vi "FPGA Main.vi"() -> ()   [LabVIEW 2015]
uses:
  Type/_RW Status.ctl
  Type/_LED States.ctl
  Type/_FPGA States.ctl
  <vilib>/Platform/TimedLoop/XDataNode/timing_clust.ctl
  <vilib>/Platform/TimedLoop/XDataNode/nitl_modes.ctl
  <vilib>/Platform/TimedLoop/XDataNode/wakeup.ctl
  Type/_FPGA DC Lines.ctl
  <vilib>/rvi/Emulation/niFpgaGetClockAttributes.vi
  <vilib>/rvi/Emulation/niFpgaSctlEmulationGetInTimedLoop.vi
  <vilib>/rvi/Emulation/niFpgaEmulationReportErrorSimple.vi
  <vilib>/rvi/eio/common/nirviEmuTemplateMethod_errors.vi
  <vilib>/rvi/Emulation/niFpgaCriticalErrorInLSC.vi
  <vilib>/rvi/Emulation/niFpgaEmulationIsFPGAContextNoSignature.vi
  <vilib>/rvi/DataTransferAndStorage/Container/Common/niFpgaContainerGetUniqueNameForEmu.vi
  <vilib>/rvi/Memory/Memory_Emulation/niFpgaMemoryEmulationCacheClearOnFirstRun.vi
  <vilib>/rvi/Memory/Memory_Emulation/nirvimemoryEmulationManagerCache_MakeExclusive.vi
  <vilib>/rvi/Memory/Memory_Emulation/niFpgaMemoryEmulationValidateCache.vi
  <vilib>/rvi/Memory/Memory_Emulation/nirvimemoryEmulationManagerCache_InsertValue.vi
  <vilib>/Utility/error.llb/Clear Errors.vi
  <vilib>/rvi/Memory/Memory_Emulation/nirvimemoryEmulationManagerCache_ReleaseExclusive.vi
  <vilib>/rvi/Memory/Memory_Emulation/nirvimemoryEmulationManagerCache_GetValue.vi
  <vilib>/rvi/Memory/Memory_Emulation/nirvimemoryEmulationManagerCache_SetValue.vi
  <vilib>/rvi/Emulation/niFpgaProcessEmulError.vi
  <vilib>/rvi/Memory/Memory_Emulation/nirvimemoryEmulation.vi
  <vilib>/rvi/Memory/Memory_Emulation/nirvimemoryFastEmulation.vi
  <vilib>/rvi/Emulation/niFpgaSctlEmulationResourceMgr.vi
  <vilib>/rvi/errors/nirviReportUnexpectedCaseInternalError (U32).vi
  Instance           1 17Saved   FPGA Main .vi
  Instance           2 17Saved   FPGA Main .vi
  <vilib>/rvi/interface/RandomDataEmulation/niFpgaRandomDataHandleErrors.vi
  <vilib>/eio/EIONode/EIONode.xnode
  <vilib>/Platform/TimedLoop/XDataNode/XDataNode.xnode
  <vilib>/rvi/DataTransferAndStorage/Container/XNode/niFpgaContainer.xnode
  <vilib>/rvi/DataTransferAndStorage/Register/Emulation/niFpgaRegisterEmulation.vi
  <vilib>/rvi/interface/RandomDataEmulation/nirviRandomDataFpgaReadWriteTemplate.vi
  <vilib>/Platform/TimedLoop/XDataNode/XDNodeRunTimeDep.lvlib
panel:
  out "i":i32
  out "Run Mode":u8
  out "FPGA States":T1
  out "Acquiring Data":bool
  out "Ready to Acquire Data":bool
  out "LC Input Detected":bool
  out "Run In Progress":bool
  in  "ForceStart":bool
  in  "FilaB":bool
  in  "FilaC":bool
  in  "Send Serial":bool
  in  "Repeat":bool
  in  "LED States":T2
  in  "Update":bool
  out "Version":u32
  in  "R/W Status":T3
  in  "Start":bool
  out "Running":bool
  in  "Address":u16
  in  "Data":u32
  in  "Read/Write":bool
  # "Memory Map Access"
  # "Run Cycle Control"
  # "VG Filament Control"
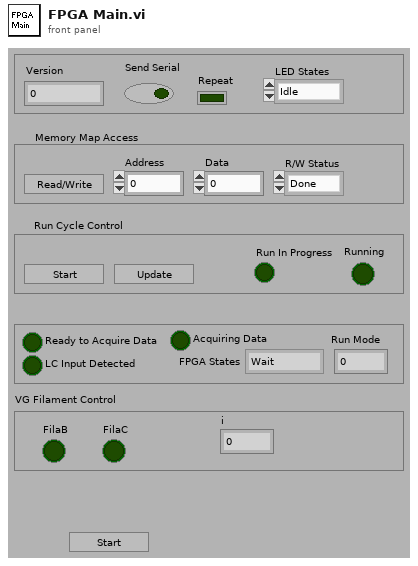
[diagram p1: front panel]
types:
  T1 = typedef "_FPGA States.ctl" = enum8{"Wait", "Single", "Dual", "DoCycles", "RampParam", "ReadADC", "SetOscil", "SetPIC", "EleOn", "Stop"}
  T2 = typedef "_LED States.ctl" = enum8{"Idle", "Solid B", "Solid R", "Solid P", "Off B", "Off R", "Off P", "Off BRP", "Off RP", "Flash R&P", "Flash P"}
  T3 = typedef "_RW Status.ctl" = enum8{"Done", "Do Read", "Do Write", "Set Latch1", "Set Latch2", "Set Latch3", "Set Latch4", "RP ON", "EL ON", "Serial Send", "Set LC Out", "Get LC In", "Read VAC", "Table Test", "Get Interlock", "Do Read2", "Do Write2"}
  T4 = typedef "_FPGA DC Lines.ctl" = enum16{"Q1 POL", "Q3 POL", "Q1 DC EN", "Q3 DC EN", "COR POL", "CUR POL", "S1 POL", "S2 POL", "CEM POL"}
  T5 = typedef "XDNodeRunTimeDep.lvlib/timing_clust.ctl" = cluster{"Expected End [f-1]":u64, "Actual End [f-1]":u64, "Finished Late? [f-1]":bool, "Expected End [i-1]":u64, "Actual End [i-1]":u64, "Finished Late? [i-1]":bool, "Expected Start [i]":u64, "Actual Start [i]":u64, "Expected Start [f]":u64, "Actual Start [f]":u64, "Source Name":string, "Structure Name":string, "Period":i64, "Deadline":i64, "Offset":i64, "Start":i64, "Priority":i32, "Timeout":i32, "Mode":T6, "Wakeup Reason":T7, "Error":errorcluster, "Source Type":string, "Secondary Source Type":string, "Global End Time":u64, "Global Start Time":u64, "Frame Duration":u64, "Iteration Duration":u64, "Assigned CPU":i32, "I/O Scan Engine Mode":u32}
  T6 = typedef "XDNodeRunTimeDep.lvlib/nitl_modes.ctl" = enum32{"No Change", "Process missed periods, maintain original phase", "Discard missed periods, maintain original phase", "Process missed periods, ignore original phase", "Discard missed periods, ignore original phase"}
  T7 = typedef "XDNodeRunTimeDep.lvlib/wakeup.ctl" = enum32{"Normal", "Aborted", "Asynchronous wakeup", "Timing source error", "Timed loop error", "Timeout"}
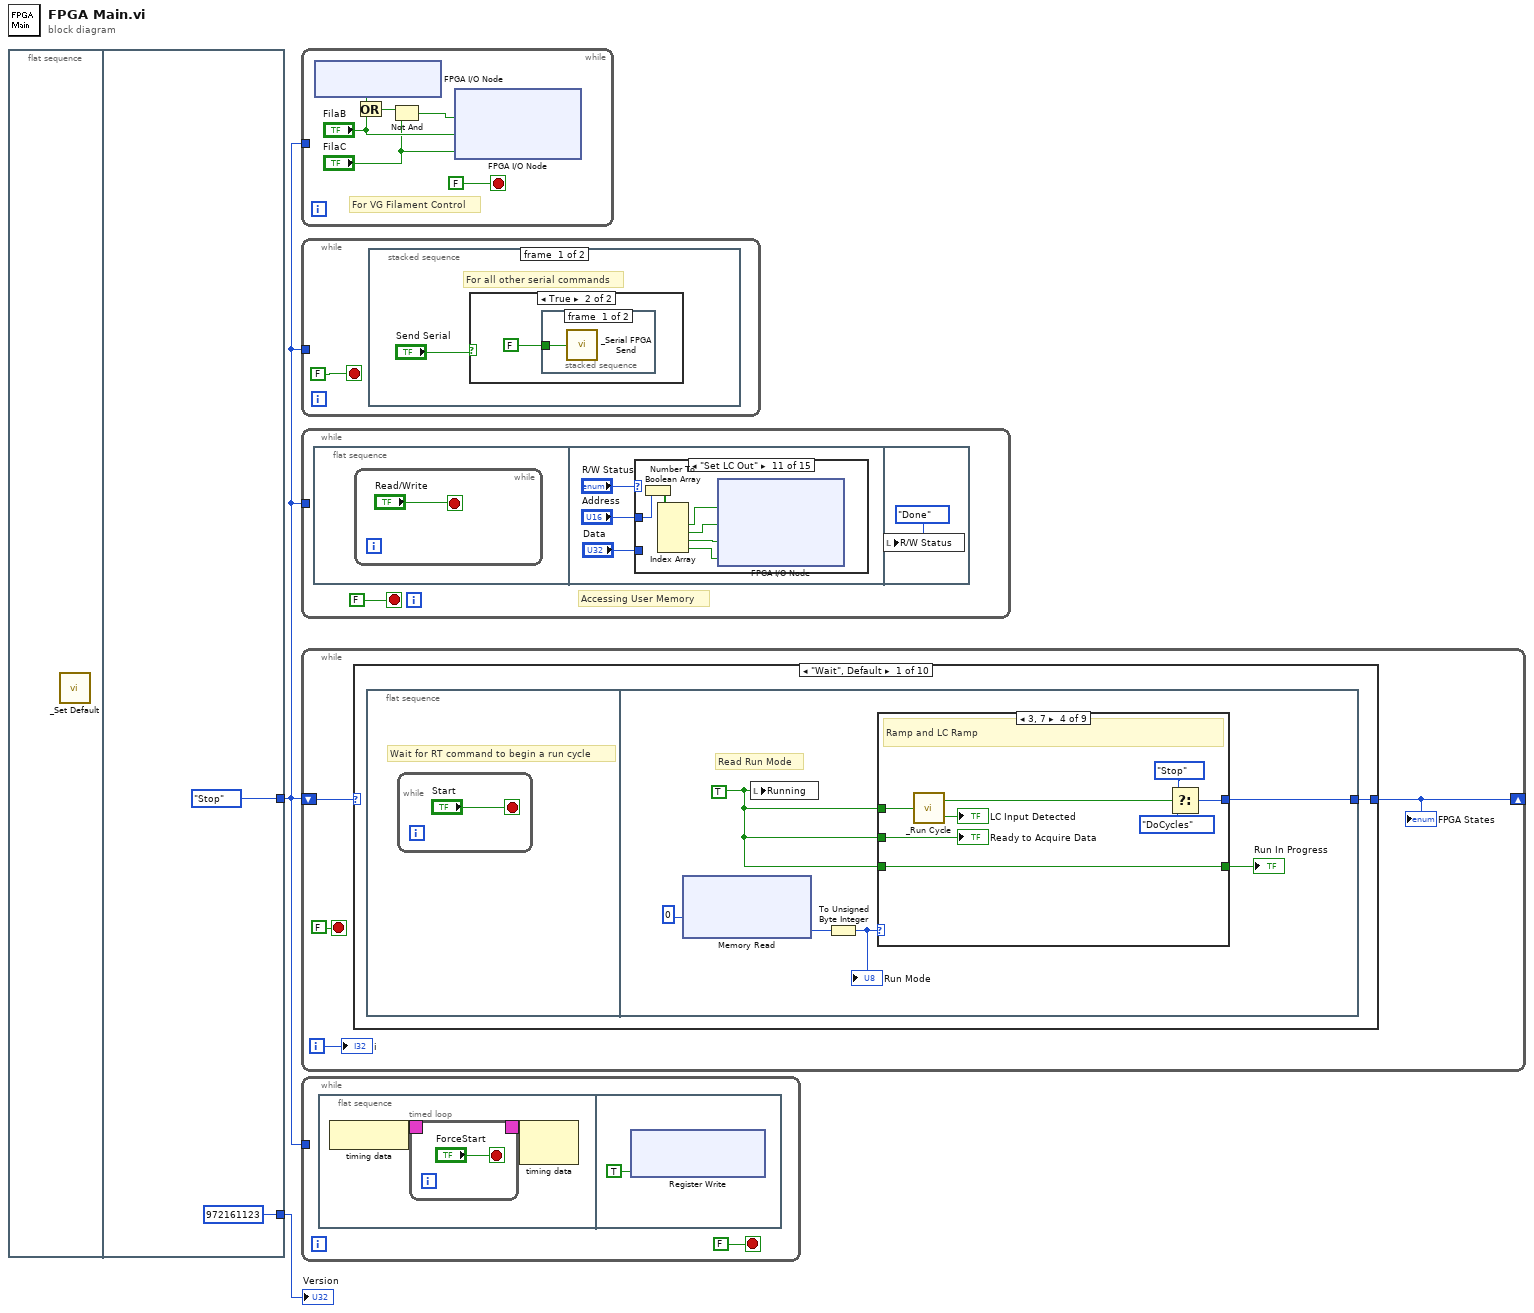
[diagram p0: block diagram]
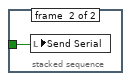
[diagram p3: hidden frame]
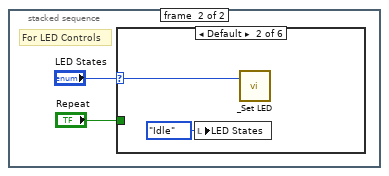
[diagram p4: hidden frame]
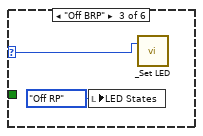
[diagram p6: hidden frame]
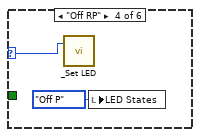
[diagram p7: hidden frame]
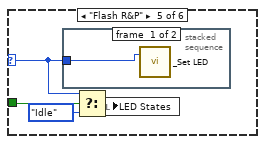
[diagram p8: hidden frame]
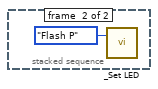
[diagram p9: hidden frame]
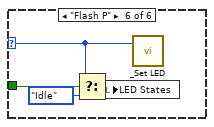
[diagram p10: hidden frame]
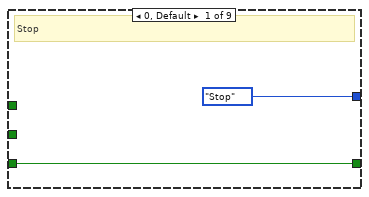
[diagram p11: hidden frame]
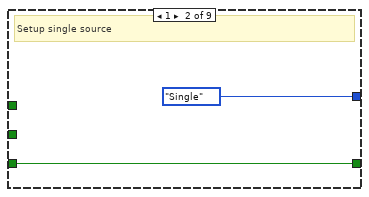
[diagram p12: hidden frame]
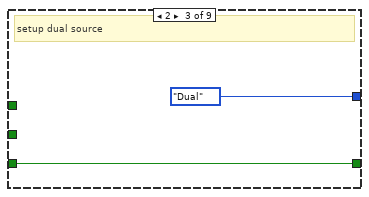
[diagram p13: hidden frame]
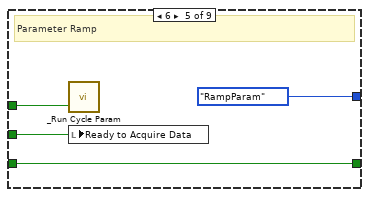
[diagram p14: hidden frame]
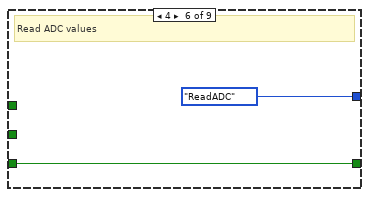
[diagram p15: hidden frame]
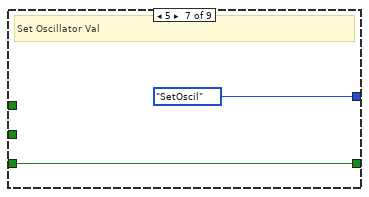
[diagram p16: hidden frame]
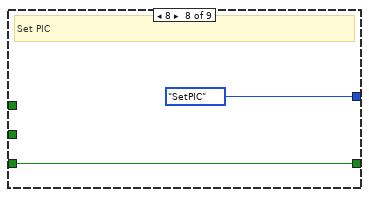
[diagram p17: hidden frame]
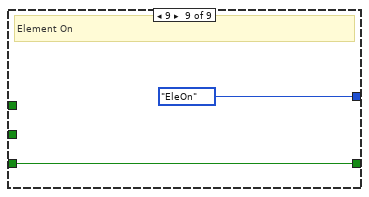
[diagram p18: hidden frame]
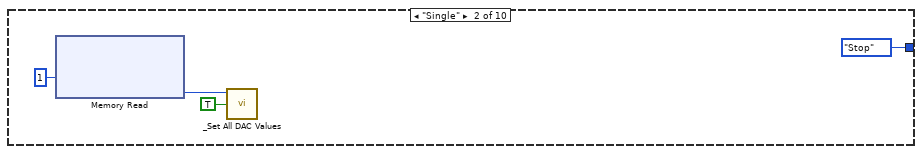
[diagram p19: hidden frame]
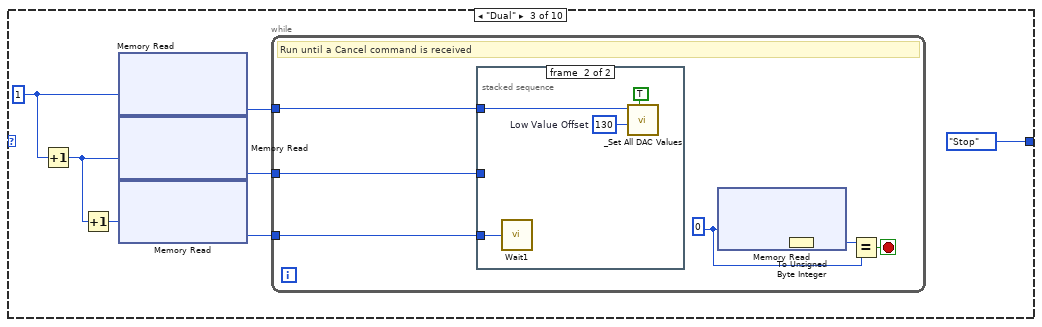
[diagram p20: hidden frame]
diagram:
  n1 = flat-sequence {
    tunnel: [_FPGA_States."Stop" ("FPGA States")] -> w2
    tunnel: [u32 972161123 ("Version")] -> w1
    frame #0 {
      n2 = call "_Set Default.vi"() -> ()  [unwired: 6 out]
    }
    frame #1 {
    }
  }
  n3 = while {
    tunnel: w2 -> [_]
    stop <- FALSE stop-if-true
    # "For VG Filament Control"
    n4 = xnode "FPGA I/O Node"() -> ("Digtal IO/DIO65"=w9:bool)  [unwired: 1 in, 1 out]
    n5 = Or(x=w9, y="FilaB") -> (x .or. y?=w8:bool)
    n6 = Not And(1:"FilaC", 2:w8) -> (0:w7:bool)
    n7 = xnode "FPGA I/O Node"("Digtal IO/DIO68"=w7, "Digtal IO/DIO66"="FilaB", "Digtal IO/DIO67"="FilaC") -> ()  [unwired: 3 in, 3 out]
  }
  n8 = while {
    tunnel: w2 -> [_]
    stop <- FALSE stop-if-true
    n9 = stacked-sequence {
      frame #0 {
        # "For all other serial commands"
        n10 = case shown="True" "Send Serial" {
          frame False {
          }
          frame True {
            n11 = stacked-sequence {
              tunnel: FALSE ("LED Control (T)") -> [w14 w15]
              frame #0 {
                n12 = call "_Serial FPGA Send.vi"("LED Control (T)"=w14) -> ()
              }
              frame #1 {
                n13 = local write "Send Serial"(w15) -> ()
              }
            }
          }
        }
      }
      frame #1 {
        # "For LED Controls"
        n14 = case shown="Default" "LED States" {
          selector: "LED States" -> [_ w18 w20 w22 w24 w30]
          tunnel: "Repeat" -> [_ _ _ _ w27 w33]
          frame "Idle" {
          }
          frame Default {
            n15 = local write "LED States"(_LED_States."Idle" ("LED States")) -> ()
            n16 = call "_Set LED.vi"("LED States"=w18) -> ()  [unwired: 3 out]
          }
          frame "Off BRP" {
            n17 = local write "LED States"(_LED_States."Off RP" ("LED States")) -> ()
            n18 = call "_Set LED.vi"("LED States"=w20) -> ()  [unwired: 3 out]
          }
          frame "Off RP" {
            n19 = call "_Set LED.vi"("LED States"=w22) -> ()  [unwired: 3 out]
            n20 = local write "LED States"(_LED_States."Off P" ("LED States")) -> ()
          }
          frame "Flash R&P" {
            n21 = stacked-sequence {
              tunnel: w24 -> [w28 _]
              frame #0 {
                n22 = call "_Set LED.vi"("LED States"=w28) -> ()  [unwired: 3 out]
              }
              frame #1 {
                n23 = call "_Set LED.vi"("LED States"=_LED_States."Flash P") -> ()  [unwired: 3 out]
              }
            }
            n24 = Select(t=w24, s=w27, f=_LED_States."Idle") -> (s? t:f=w26:T2)
            n25 = local write "LED States"(w26) -> ()
          }
          frame "Flash P" {
            n26 = Select(t=w30, s=w33, f=_LED_States."Idle") -> (s? t:f=w32:T2)
            n27 = local write "LED States"(w32) -> ()
            n28 = call "_Set LED.vi"("LED States"=w30) -> ()  [unwired: 3 out]
          }
        }
      }
    }
  }
  n29 = while {
    tunnel: w2 -> [_]
    stop <- FALSE stop-if-true
    # "Accessing User Memory"
    n30 = flat-sequence {
      frame #0 {
        n31 = while {
          stop <- "Read/Write" stop-if-true
        }
      }
      frame #1 {
        n32 = case shown="\"Set LC Out\"" "R/W Status" {
          tunnel: "Address" -> [_ w39 w42 w44 w46 w47 w49 w51 w53 w55 w61 _ _ _ _]
          tunnel: "Data" -> [_ _ _ w43 w45 _ _ _ _ _ _ _ _ _ _]
          frame "Done", Default {
          }
          frame "Do Read" {
            n33 = xnode ("Memory Read")("Address"=w39) -> ("Data"=w40:u32)  [unwired: 1 in, 1 out]
            n34 = local write "Data"(w40) -> ()
          }
          frame "Do Read2" {
            n35 = xnode ("Memory Read")("Address"=w42) -> ("Data"=w41:u32)  [unwired: 1 in, 1 out]
            n36 = local write "Data"(w41) -> ()
          }
          frame "Do Write" {
            n37 = xnode ("Memory Write")("Address"=w44, "Data"=w43) -> ()  [unwired: 1 in, 1 out]
          }
          frame "Do Write2" {
            n38 = xnode ("Memory Write")("Address"=w46, "Data"=w45) -> ()  [unwired: 1 in, 1 out]
          }
          frame "Set Latch1" {
            n39 = call "_Set DC Line.vi"("States"=w47, "DC Line"=_FPGA_DC_Lines."Q1 POL") -> ()  [unwired: 2 out]
          }
          frame "Set Latch2" {
            n40 = call "_Set DC Line.vi"("States"=w49, "DC Line"=_FPGA_DC_Lines."COR POL") -> ()  [unwired: 2 out]
          }
          frame "Set Latch3" {
            n41 = call "_Set DC Line.vi"("States"=w51, "DC Line"=_FPGA_DC_Lines."S1 POL") -> ()  [unwired: 2 out]
          }
          frame "Set Latch4" {
            n42 = call "_Set DC Line.vi"("States"=w53, "DC Line"=_FPGA_DC_Lines."CEM POL") -> ()  [unwired: 2 out]
          }
          frame "RP ON" {
            n43 = Greater Than 0?(x=w55) -> (x > 0?=w56:bool)
            n44 = xnode "FPGA I/O Node"("Digtal IO/DIO18"=w56) -> ()  [unwired: 1 in, 1 out]
          }
          frame "Set LC Out" {
            n45 = Number To Boolean Array(number=w61) -> (Boolean array=w62:bool[])
            n46 = Index Array(array=w62) -> (element #1=w60:bool, element #2=w59:bool, element #3=w58:bool, element #4=w57:bool)  [unwired: 4 in]
            n47 = xnode "FPGA I/O Node"("Digtal IO/DIO49"=w60, "Digtal IO/DIO50"=w59, "Digtal IO/DIO52"=w58, "Digtal IO/DIO56"=w57) -> ()  [unwired: 4 in, 4 out]
          }
          frame "Get LC In" {
            # "LC2-I1"
            # "LC1-I1"
            n48 = xnode "FPGA I/O Node"() -> ("Digtal IO/DIO51"=w67:bool, "Digtal IO/DIO53"=w66:bool)  [unwired: 2 in, 2 out]
            n49 = Boolean To (0,1)(Boolean=w66) -> (0, 1=w64:i16)
            n50 = Boolean To (0,1)(Boolean=w67) -> (0, 1=w65:i16)
            n51 = Join Numbers(hi=w65, lo=w64) -> ((hi.lo)=w63:u32)
            n52 = local write "Data"(w63) -> ()
          }
          frame "Get Interlock" {
            # "Card cage door"
            n53 = xnode "FPGA I/O Node"() -> ("Digtal IO/DIO60"=w69:bool)  [unwired: 1 in, 1 out]
            n54 = Boolean To (0,1)(Boolean=w69) -> (0, 1=w68:i16)
            n55 = local write "Data"(w68) -> ()
          }
          frame "Read VAC" {
            n56 = call "_Read VAC Gauge.vi"() -> ("DAC"=w70:u8)
            n57 = local write "Data"(w70) -> ()
          }
          frame "Table Test" {
            n58 = call "_Table Test.vi"() -> ()  [unwired: 1 out]
          }
        }
      }
      frame #2 {
        n59 = local write "R/W Status"(_RW_Status."Done" ("RW Status")) -> ()
      }
    }
  }
  n60 = while {
    shift-right: [w74] -> _
    shift-left: w2 -> [w75]
    i -> [w72]
    stop <- FALSE stop-if-true
    n61 = case shown="\"Wait\", Default" w75 {
      tunnel: [w76 _FPGA_States."Stop" ("FPGA States") _FPGA_States."Stop" ("FPGA States") _FPGA_States."Stop" ("FPGA States") _FPGA_States."Stop" ("FPGA States") _FPGA_States."Stop" ("FPGA States") _FPGA_States."Stop" ("FPGA States") _FPGA_States."Stop" ("FPGA States") _FPGA_States."Stop" ("FPGA States") _FPGA_States."Wait" ("FPGA States")] -> w74
      frame "Wait", Default {
        n62 = flat-sequence {
          tunnel: [w83] -> w76
          frame #0 {
            # "Wait for RT command to begin a run cycle"
            n63 = while {
              stop <- "Start" stop-if-true
            }
          }
          frame #1 {
            w78 = TRUE ("Running")
            # "Read Run Mode"
            n64 = xnode ("Memory Read")("Address"=u8 0) -> ("Data"=w82:u32)  [unwired: 1 in, 1 out]
            n65 = local write "Running"(w78) -> ()
            n66 = To Unsigned Byte Integer(number=w82) -> (unsigned 8bit integer=w80:u8)
            "Run Mode" <- w80
            n67 = case shown="3, 7" w80 {
              tunnel: [_FPGA_States."Stop" ("FPGA States") _FPGA_States."Single" ("FPGA States") _FPGA_States."Dual" ("FPGA States") w94 _FPGA_States."RampParam" ("FPGA States") _FPGA_States."ReadADC" ("FPGA States") _FPGA_States."SetOscil" ("FPGA States") _FPGA_States."SetPIC" ("FPGA States") _FPGA_States."EleOn" ("FPGA States")] -> w83
              tunnel: w78 -> [_ _ _ w93 w100 _ _ _ _]
              tunnel: [w84 w86 w88 w92 w99 w102 w104 w106 w108] -> w79
              tunnel: w78 -> [w84 w86 w88 w92 w99 w102 w104 w106 w108]
              tunnel: w78 -> [_ _ _ w90 w98 _ _ _ _]
              frame 0, Default {
                # "Stop"
              }
              frame 1 {
                # "Setup single source"
              }
              frame 2 {
                # "setup dual source"
              }
              frame 3, 7 {
                # "Ramp and LC Ramp"
                n68 = call "_Run Cycle.vi"("Init (F)"=w93) -> ("LC Input Detected"=→"LC Input Detected":bool, "Finish Run?"=w97:bool)  [unwired: 2 in]
                n69 = Select(t=_FPGA_States."Stop" ("FPGA States"), s=w97, f=_FPGA_States."DoCycles" ("FPGA States")) -> (s? t:f=w94:T1)
                "Ready to Acquire Data" <- w90
              }
              frame 6 {
                # "Parameter Ramp"
                n70 = call "_Run Cycle Param.vi"("Init (F)"=w100) -> ()  [unwired: 2 out]
                n71 = local write "Ready to Acquire Data"(w98) -> ()
              }
              frame 4 {
                # "Read ADC values"
              }
              frame 5 {
                # "Set Oscillator Val"
              }
              frame 8 {
                # "Set PIC"
              }
              frame 9 {
                # "Element On"
              }
            }
            "Run In Progress" <- w79
          }
        }
      }
      frame "Single" {
        n72 = xnode ("Memory Read")("Address"=u32 1) -> ("Data"=w112:u32)  [unwired: 1 in, 1 out]
        n73 = call "_Set All DAC Values.vi"("Record Values (F)"=TRUE, "# of Active Channels"=w112) -> ()  [unwired: 7 in]
      }
      frame "Dual" {
        w116 = u8 1 ("Address")
        n74 = Increment(x=w116) -> (x+1=w114:u8)
        n75 = Increment(x=w114) -> (x+1=w115:u8)
        n76 = xnode ("Memory Read")("Address"=w116) -> ("Data"=w119:u32)  [unwired: 1 in, 1 out]
        n77 = xnode ("Memory Read")("Address"=w114) -> ("Data"=w118:u32)  [unwired: 1 in, 1 out]
        n78 = xnode ("Memory Read")("Address"=w115) -> ("Data"=w117:u32)  [unwired: 1 in, 1 out]
        n79 = while {
          tunnel: w118 -> [w127]
          tunnel: w117 -> [w126]
          tunnel: w119 -> [w125]
          stop <- w122 stop-if-true
          w121 = u8 0 ("Address")
          # "Run until a Cancel command is received"
          n80 = stacked-sequence {
            tunnel: w127 -> [w130 _]
            tunnel: w126 -> [_ w133]
            tunnel: w125 -> [w129 w132]
            frame #0 {
              n81 = call "Wait"("Count(uSec)"=w130) -> ()  [unwired: 1 out]
              n82 = call "_Set All DAC Values.vi"("Record Values (F)"=TRUE, "# of Active Channels"=w129) -> ()  [unwired: 7 in]
            }
            frame #1 {
              w134 = u16 130  # Low Value Offset
              n83 = call "Wait1"("Count(uSec)"=w133) -> ()  [unwired: 1 out]
              n84 = call "_Set All DAC Values.vi"("Record Values (F)"=TRUE, "DAC Value Offset (70)"=w134, "# of Active Channels"=w132) -> ()  [unwired: 6 in]
            }
          }
          n85 = xnode ("Memory Read")("Address"=w121) -> ("Data"=w124:u32)  [unwired: 1 in, 1 out]
          n86 = To Unsigned Byte Integer(number=w124) -> (unsigned 8bit integer=w123:u8)
          n87 = Equal?(x=w123, y=w121) -> (x = y?=w122:bool)
        }
      }
      frame "DoCycles" {
        n88 = flat-sequence {
          frame #0 {
            # "Run Cycle"
            n89 = while {
              tunnel: [w142] -> w138
              i -> [w142]
              stop <- w140 stop-if-true
              n90 = call "_Run Cycle.vi"("Update"="Update") -> ("Finish Run?"=w140:bool)  [unwired: 1 in, 2 out]
            }
            n91 = To Unsigned Long Integer(number=w138) -> (unsigned 32bit integer=w137:u32)
            n92 = xnode ("Memory Write")("Address"=u32 7, "Data"=w137) -> ()  [unwired: 1 in, 1 out]
          }
          frame #1 {
            # "Signaling the end of Run"
            n93 = xnode ("FIFO Write")("Element"=-2147483648, "Timeout"=u8 50 ("Timeout (-1 for no timeout)")) -> ()  [unwired: 1 in, 2 out]
            n94 = call "_Set All DAC Values.vi"("DAC Value Offset (70)"=u16 394, "Channel ID Offset (10)"=u16 390, "# of Active Channels"=u16 4) -> ()  [unwired: 6 in]
          }
          frame #2 {
            # "Turn off LC Stop"
            n95 = call "_Update LC Out.vi"("LC Stop"=FALSE, "LC Hold"=TRUE) -> ()  [unwired: 6 out]
          }
        }
        "Acquiring Data" <- TRUE ("Acquiring Data")
      }
      frame "RampParam" {
        n96 = flat-sequence {
          frame #0 {
            # "Run Parameter Ramp"
            n97 = while {
              tunnel: [w159] -> w153
              i -> [w159]
              stop <- w160 stop-if-true
              w156 = u8 0 ("Address")
              n98 = xnode ("Memory Read")("Address"=w156) -> ("Data"=w158:u32)  [unwired: 1 in, 1 out]
              n99 = call "_Run Cycle Param.vi"() -> ("Finish Run?"=w161:bool)  [unwired: 1 in, 1 out]
              n100 = To Unsigned Byte Integer(number=w158) -> (unsigned 8bit integer=w157:u8)
              n101 = Equal?(x=w157, y=w156) -> (x = y?=w155:bool)
              n102 = Or(x=w161, y=w155) -> (x .or. y?=w160:bool)
            }
            n103 = To Unsigned Long Integer(number=w153) -> (unsigned 32bit integer=w152:u32)
            n104 = xnode ("Memory Write")("Address"=u32 7, "Data"=w152) -> ()  [unwired: 1 in, 1 out]
          }
          frame #1 {
            # "Signaling the end of Run"
            n105 = xnode ("FIFO Write")("Element"=-2147483648, "Timeout"=u8 50 ("Timeout (-1 for no timeout)")) -> ()  [unwired: 1 in, 2 out]
            n106 = call "_Set All DAC Values.vi"("DAC Value Offset (70)"=u16 394, "Channel ID Offset (10)"=u16 390, "# of Active Channels"=u16 4) -> ()  [unwired: 6 in]
          }
          frame #2 {
            # "Turn off LC Stop"
            n107 = call "_Update LC Out.vi"("LC Stop"=FALSE, "LC Hold"=TRUE) -> ()  [unwired: 6 out]
          }
        }
        n108 = local write "Acquiring Data"(TRUE ("Acquiring Data")) -> ()
      }
      frame "ReadADC" {
        n109 = for {
          N: u8 128 -> [_]
          i -> [w172]
          # "Read all ADC Values"
          n110 = To Byte Integer(number=w172) -> (8bit integer=w171:i8)
          n111 = call "_Read ADC.vi"("Channel #"=w171) -> ()  [unwired: 1 out]
        }
      }
      frame "SetOscil" {
        n112 = call "_Set Oscillator.vi"() -> ()  [unwired: 2 out]
      }
      frame "SetPIC" {
        w177 = u32 7 ("Address")
        n113 = Increment(x=w177) -> (x+1=w176:u32)
        n114 = xnode ("Memory Read")("Address"=w177) -> ("Data"=w175:u32)  [unwired: 1 in, 1 out]
        n115 = xnode ("Memory Read")("Address"=w176) -> ("Data"=w174:u32)  [unwired: 1 in, 1 out]
        n116 = call "_Set 1 DAC Value.vi"("DAC"=w174, "Ch#"=w175) -> ()  [unwired: 2 out]
      }
      frame "EleOn" {
        n117 = call "_Electronic On.vi"() -> ()  [unwired: 1 out]
      }
      frame "Stop" {
        n118 = flat-sequence {
          frame #0 {
            n119 = call "_Chip Select.vi"() -> ()  [unwired: 1 in, 7 out]
          }
          frame #1 {
            n120 = call "_Update Serial DAC.vi"() -> ()  [unwired: 4 in, 4 out]
          }
          frame #2 {
            w181 = FALSE
            n121 = xnode ("Register Write")("Data"=w181) -> ()  [unwired: 1 in, 1 out]
            n122 = local write "Run In Progress"(w181) -> ()
            n123 = local write "Ready to Acquire Data"(w181) -> ()
            n124 = local write "LC Input Detected"(w181) -> ()
            n125 = local write "Acquiring Data"(w181) -> ()
            "Running" <- w181
          }
        }
      }
    }
    "FPGA States" <- w74
    "i" <- w72
  }
  n126 = while {
    tunnel: w2 -> [_]
    stop <- FALSE stop-if-true
    n127 = flat-sequence {
      frame #0 {
        n128 = node-c288() -> (w184:T5)
        n129 = timed-loop {
          timing-out: [_] -> w183
          timing: w184 -> [_]
          stop <- "ForceStart" stop-if-true
        }
        n130 = node-c288(w183) -> ()  [unwired: 1 out]
      }
      frame #1 {
        n131 = xnode ("Register Write")("Data"=TRUE) -> ()  [unwired: 1 in, 1 out]
      }
    }
  }
  "Version" <- w1
